vi "Initialize pressure boxes 32bit.vi"(11 "Number of \nPressure Boxes":i32) -> (1 "error out Box ID2":errorcluster, 2 "error out Box ID1":errorcluster, 3 "error out Box ID0":errorcluster)   [LabVIEW 2014]
uses:
  Automation/PacDrive/PacDrive.dll
panel:
  in  "error in Box ID2":errorcluster
  in  "error in Box ID1":errorcluster
  in  "error in Box ID0":errorcluster
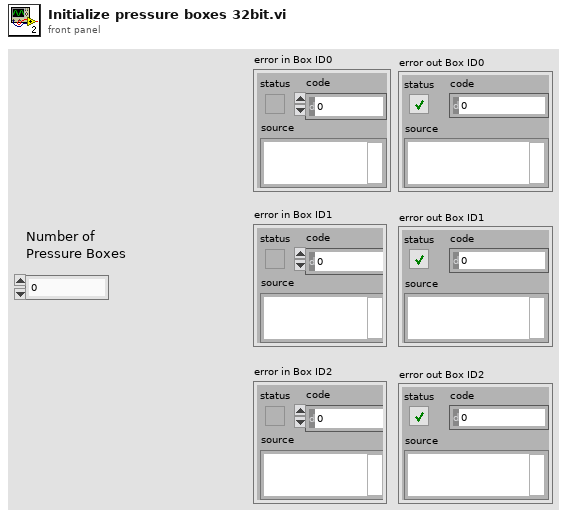
[diagram p1: front panel]
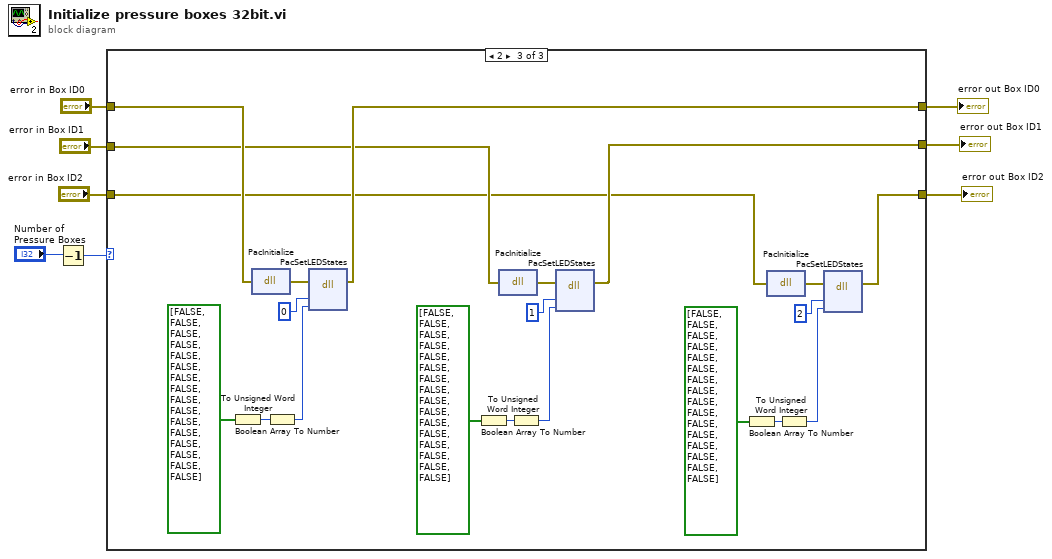
[diagram p0: block diagram]
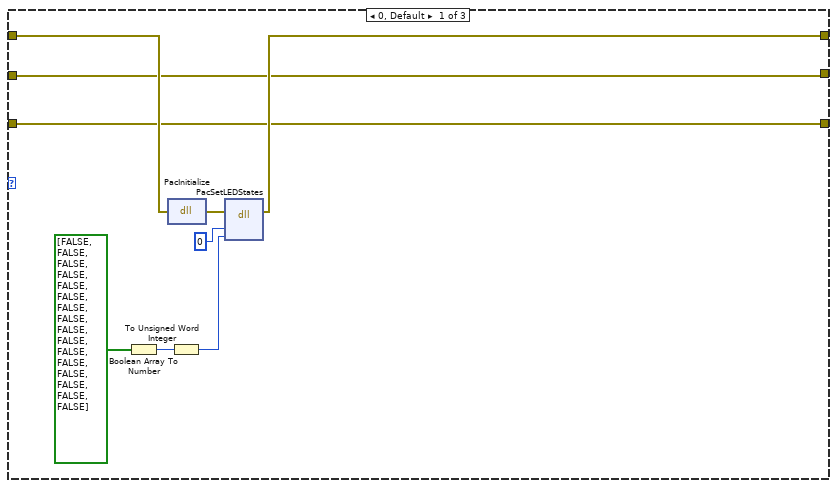
[diagram p2: hidden frame]
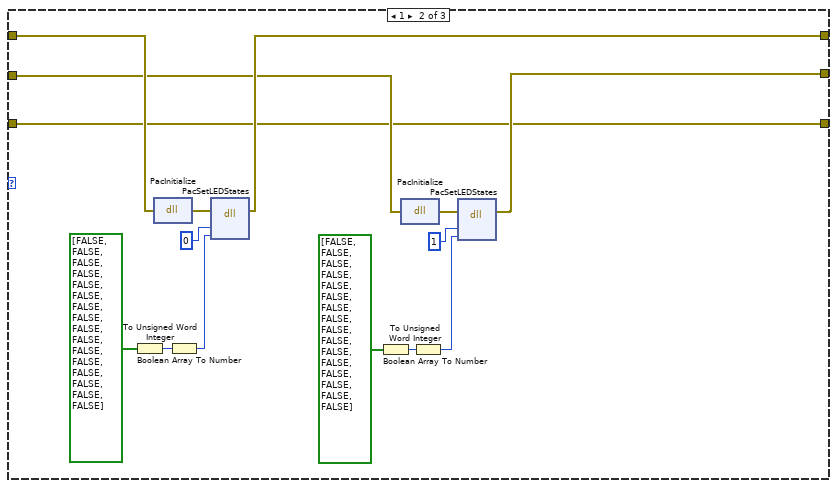
[diagram p3: hidden frame]
diagram:
  n1 = Decrement(x="Number of \nPressure Boxes") -> (x-1=w2:i32)
  n2 = case shown="2" w2 {
    tunnel: "error in Box ID0" -> [w12 w27 w48]
    tunnel: "error in Box ID1" -> [w10 w20 w41]
    tunnel: "error in Box ID2" -> [w9 w18 w34]
    tunnel: [w11 w26 w47] -> w5
    tunnel: [w10 w19 w40] -> w4
    tunnel: [w9 w18 w33] -> w3
    frame 0, Default {
      n3 = Boolean Array To Number(Boolean array=bool[] [FALSE, FALSE, FALSE, FALSE, FALSE, FALSE, FALSE, FALSE, FALSE, FALSE, FALSE, FALSE, FALSE, FALSE, FALSE, FALSE]) -> (number=w16:u32)
      n4 = dll-call lib="I:/Transfer/Marija/Automation/PacDrive/PacDrive.dll" fn="PacInitialize"(error in=w12) -> (error out=w14:errorcluster)  [unwired: 3 in, 1 out]
      n5 = To Unsigned Word Integer(number=w16) -> (unsigned 16bit integer=w15:u16)
      n6 = dll-call lib="I:/Transfer/Marija/Automation/PacDrive/PacDrive.dll" fn="PacSetLEDStates"(error in=w14, "PacNum"=0, "LEDStates"=w15) -> (error out=w11:errorcluster)  [unwired: 5 in, 1 out]
    }
    frame 1 {
      n7 = Boolean Array To Number(Boolean array=bool[] [FALSE, FALSE, FALSE, FALSE, FALSE, FALSE, FALSE, FALSE, FALSE, FALSE, FALSE, FALSE, FALSE, FALSE, FALSE, FALSE]) -> (number=w29:u32)
      n8 = dll-call lib="I:/Transfer/Marija/Automation/PacDrive/PacDrive.dll" fn="PacInitialize"(error in=w27) -> (error out=w31:errorcluster)  [unwired: 3 in, 1 out]
      n9 = To Unsigned Word Integer(number=w29) -> (unsigned 16bit integer=w30:u16)
      n10 = dll-call lib="I:/Transfer/Marija/Automation/PacDrive/PacDrive.dll" fn="PacSetLEDStates"(error in=w31, "PacNum"=0, "LEDStates"=w30) -> (error out=w26:errorcluster)  [unwired: 5 in, 1 out]
      n11 = Boolean Array To Number(Boolean array=bool[] [FALSE, FALSE, FALSE, FALSE, FALSE, FALSE, FALSE, FALSE, FALSE, FALSE, FALSE, FALSE, FALSE, FALSE, FALSE, FALSE]) -> (number=w24:u32)
      n12 = dll-call lib="I:/Transfer/Marija/Automation/PacDrive/PacDrive.dll" fn="PacInitialize"(error in=w20) -> (error out=w22:errorcluster)  [unwired: 3 in, 1 out]
      n13 = To Unsigned Word Integer(number=w24) -> (unsigned 16bit integer=w23:u16)
      n14 = dll-call lib="I:/Transfer/Marija/Automation/PacDrive/PacDrive.dll" fn="PacSetLEDStates"(error in=w22, "PacNum"=1, "LEDStates"=w23) -> (error out=w19:errorcluster)  [unwired: 5 in, 1 out]
    }
    frame 2 {
      n15 = Boolean Array To Number(Boolean array=bool[] [FALSE, FALSE, FALSE, FALSE, FALSE, FALSE, FALSE, FALSE, FALSE, FALSE, FALSE, FALSE, FALSE, FALSE, FALSE, FALSE]) -> (number=w50:u32)
      n16 = dll-call lib="I:/Transfer/Marija/Automation/PacDrive/PacDrive.dll" fn="PacInitialize"(error in=w48) -> (error out=w52:errorcluster)  [unwired: 3 in, 1 out]
      n17 = To Unsigned Word Integer(number=w50) -> (unsigned 16bit integer=w51:u16)
      n18 = dll-call lib="I:/Transfer/Marija/Automation/PacDrive/PacDrive.dll" fn="PacSetLEDStates"(error in=w52, "PacNum"=0, "LEDStates"=w51) -> (error out=w47:errorcluster)  [unwired: 5 in, 1 out]
      n19 = Boolean Array To Number(Boolean array=bool[] [FALSE, FALSE, FALSE, FALSE, FALSE, FALSE, FALSE, FALSE, FALSE, FALSE, FALSE, FALSE, FALSE, FALSE, FALSE, FALSE]) -> (number=w45:u32)
      n20 = dll-call lib="I:/Transfer/Marija/Automation/PacDrive/PacDrive.dll" fn="PacInitialize"(error in=w41) -> (error out=w43:errorcluster)  [unwired: 3 in, 1 out]
      n21 = To Unsigned Word Integer(number=w45) -> (unsigned 16bit integer=w44:u16)
      n22 = dll-call lib="I:/Transfer/Marija/Automation/PacDrive/PacDrive.dll" fn="PacSetLEDStates"(error in=w43, "PacNum"=1, "LEDStates"=w44) -> (error out=w40:errorcluster)  [unwired: 5 in, 1 out]
      n23 = Boolean Array To Number(Boolean array=bool[] [FALSE, FALSE, FALSE, FALSE, FALSE, FALSE, FALSE, FALSE, FALSE, FALSE, FALSE, FALSE, FALSE, FALSE, FALSE, FALSE]) -> (number=w36:u32)
      n24 = dll-call lib="I:/Transfer/Marija/Automation/PacDrive/PacDrive.dll" fn="PacInitialize"(error in=w34) -> (error out=w38:errorcluster)  [unwired: 3 in, 1 out]
      n25 = To Unsigned Word Integer(number=w36) -> (unsigned 16bit integer=w37:u16)
      n26 = dll-call lib="I:/Transfer/Marija/Automation/PacDrive/PacDrive.dll" fn="PacSetLEDStates"(error in=w38, "PacNum"=2, "LEDStates"=w37) -> (error out=w33:errorcluster)  [unwired: 5 in, 1 out]
    }
  }
  "error out Box ID0" <- w5
  "error out Box ID1" <- w4
  "error out Box ID2" <- w3
